vi "SAACPTraceReadSignal.vi"(0 "instrument handle":refnum<k15>, 1 "Amplitude":dbl, 5 "RepCapIdentifier":string="ACP_Results" caption="RepCapIdentifier (ACP_Results)", 7 "MaxTime":i32 caption="MaxTime (ms)" format="%#.0f", 9 "Frequency":dbl caption="Frequency (Hz)", 11 "error in (no error)":errorcluster {"code" format="%.0x"}, 12 "RetValBufferSize":i32=2048 caption="RetValBufferSize (2048)") -> (4 "instrument handle out":refnum<k15>, 6 "RetVal":dbl[](array[numeric]) format="%.2p", 8 "RetValActualSize":i32, 15 "error out":errorcluster {"code" format="%.0x"})   [LabVIEW 2009, in "Keysight XSAn.lvlib"]
doc: "Initiates the measurement and puts valid data into the output buffer.\n\nSupported Models: M9290A, N8973B, N8974B, N8975B, N8976B, N9000A, N9000B, N9010A, N9010B, N9020A, N9020B, N9030A, N9030B, N9038A, N9040B, N9041B, SPN9003A, SPN9026A"
uses:
  <instrlib>/Keysight XSAn/Keysight XSAn.lvlib
  AgXSAn.dll
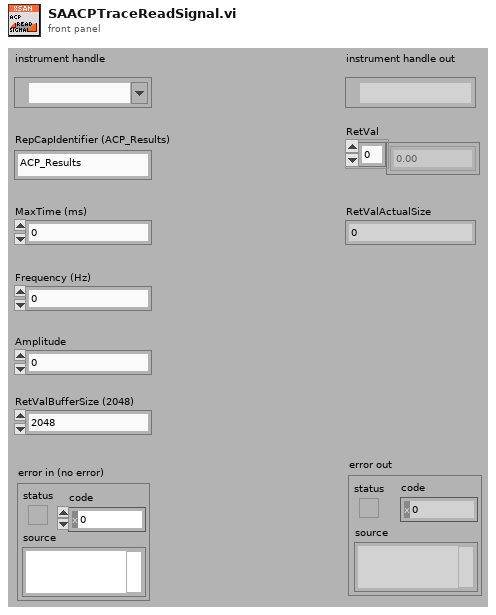
[diagram p1: front panel]
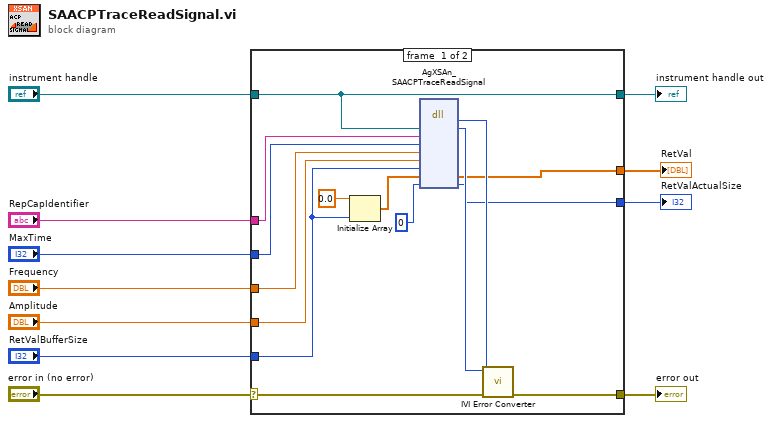
[diagram p0: block diagram]
diagram:
  n1 = case shown="No Error" "error in (no error)" {
    selector: "error in (no error)" -> [w24 w28]
    tunnel: [w23 w28] -> w11
    tunnel: "instrument handle" -> [w13 w27]
    tunnel: "RepCapIdentifier" -> [w22 _]
    tunnel: "MaxTime" -> [w21 _]
    tunnel: "Frequency" -> [w20 _]
    tunnel: "Amplitude" -> [w19 _]
    tunnel: "RetValBufferSize" -> [w12 _]
    tunnel: [w16 _] -> w3
    tunnel: [w14 _] -> w2
    tunnel: [w13 w27] -> w1
    frame #0 {
      n2 = Initialize Array(0.0 ("element"), w12) -> (w18:dbl[])
      n3 = dll-call lib="AgXSAn**.dll" fn="AgXSAn_SAACPTraceReadSignal"("Vi"=w13, "RepCapIdentifier"=w22, "MaxTime"=w21, "Frequency"=w20, "Amplitude"=w19, "RetValBufferSize"=w12, "RetVal"=w18, "RetValActualSize"=0) -> (w25:i32, "Vi"=w26:u32, "RetVal"=w16:dbl[], "RetValActualSize"=w14:i32)  [unwired: 8 in, 2 out]
      n4 = call <instrlib>:"IVI Error Converter.vi"("error in (no error)"=w24, "IVI error code (0)"=w25, "instrument handle"=w26) -> ("error out"=w23:errorcluster)  [unwired: 7 in, 1 out]
    }
    frame #1 {
    }
  }
  "error out" <- w11
  "instrument handle out" <- w1
  "RetVal" <- w3
  "RetValActualSize" <- w2
